vi "Write AO Task.vi"(6 "AOChConfigs":refnum<class "AOChConfig.lvclass">[](array[class]), 8 "error in (no error)":errorcluster, 9 "AO Waveforms":waveform(dbl)[](array[waveform]), 10 "AO DAQChannels":tag[](array[tag]), 11 "IO Device in":refnum<class "IO Device.lvclass">) -> (0 "error out":errorcluster, 3 "IO Device out":refnum<class "IO Device.lvclass">)   [LabVIEW 2015, in "IO Device.lvlib" / "IO Device.lvclass"]
uses:
  IO Device.lvclass
  Analog Output Channel/AOChConfig.lvclass
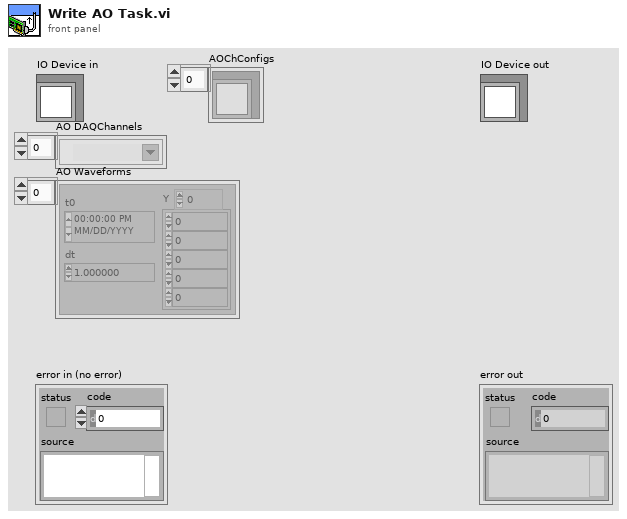
[diagram p1: front panel]
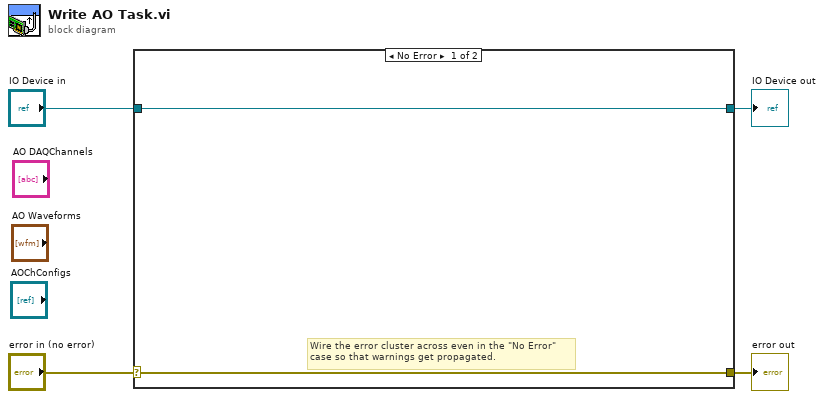
[diagram p0: block diagram]
diagram:
  n1 = case shown="No Error" "error in (no error)" {
    selector: "error in (no error)" -> [w5 w8]
    tunnel: [w5 w8] -> w3
    tunnel: [w6 w7] -> w1
    tunnel: "IO Device in" -> [w6 w7]
    frame No Error {
      # "Wire the error cluster across even in the \"No Error\"\ncase so that warnings get propagated."
    }
    frame Error {
    }
  }
  "error out" <- w3
  "IO Device out" <- w1
